vi "MListbox Clear All Rows.vi"(8 "error in (no error)":errorcluster, 11 "Multicolumn ListBox in":refnum<class "Multicolumn ListBox.lvclass">) -> (0 "error out":errorcluster, 3 "Multicolumn ListBox out":refnum<class "Multicolumn ListBox.lvclass">)   [LabVIEW 2012, in "Multicolumn ListBox.lvclass"]
uses:
  Multicolumn ListBox.lvclass
  <vilib>/Utility/miscctls.llb/LVRowAndColumnUnsignedTypeDef.ctl
  <vilib>/Utility/miscctls.llb/LVRowAndColumnTypeDef.ctl
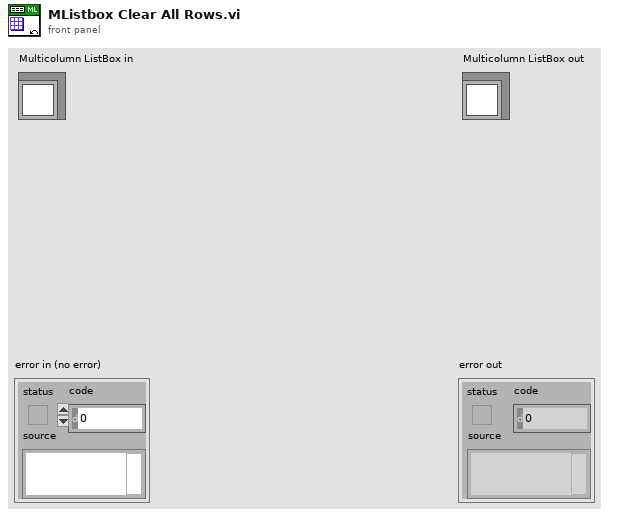
[diagram p1: front panel]
types:
  T1 = typedef "LVRowAndColumnTypeDef.ctl" = cluster{"Row":i32, "Column":i32}
  T2 = typedef "LVRowAndColumnUnsignedTypeDef.ctl" = cluster{"Row":u32, "Column":u32}
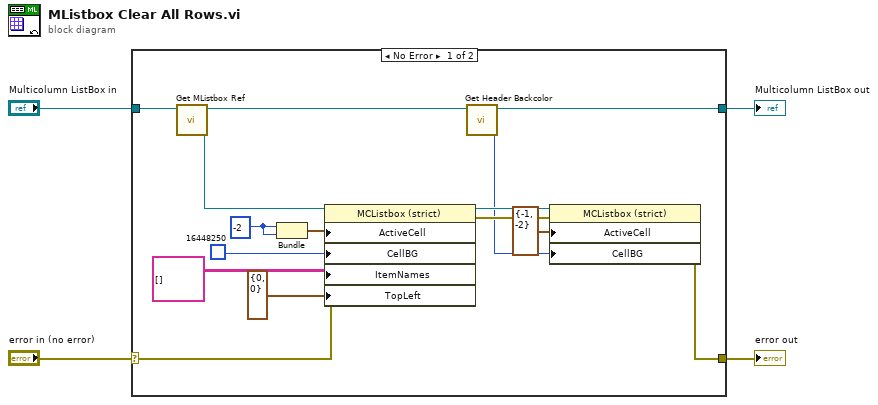
[diagram p0: block diagram]
diagram:
  n1 = case shown="No Error" "error in (no error)" {
    selector: "error in (no error)" -> [w12 w21]
    tunnel: [w7 w21] -> w3
    tunnel: [w17 w20] -> w1
    tunnel: "Multicolumn ListBox in" -> [w19 w20]
    frame No Error {
      w16 = -2
      n2 = call "Get MListbox Ref.vi"("Multicolumn ListBox in"=w19) -> ("MListbox Ref"=w13:refnum<vi>, "Multicolumn ListBox out"=w18:refnum<class "Multicolumn ListBox.lvclass">)  [unwired: 8 in, 1 out]
      n3 = Bundle(w16, w16) -> (w15:cluster{i32, i32})  [unwired: 1 in]
      n4 = property class="MCListbox (strict)"(reference=w13, error in=w12, "ActiveCell"=w15, "CellBG"=u32 16448250, "ItemNames"=string[][] [] ("Item Names"), "TopLeft"=T2 {"Row"=0, "Column"=0} ("Top Left Visible Cell")) -> (reference out=w9:refnum<vi>, error out=w8:errorcluster)
      n5 = call "Get Header Backcolor.vi"("Multicolumn ListBox in"=w18) -> ("Header Backcolor"=w6:u32, "Multicolumn ListBox out"=w17:refnum<class "Multicolumn ListBox.lvclass">)  [unwired: 8 in, 1 out]
      n6 = property class="MCListbox (strict)"(reference=w9, error in=w8, "ActiveCell"=T1 {"Row"=-1, "Column"=-2} ("Active Cell:Active Cell"), "CellBG"=w6) -> (error out=w7:errorcluster)  [unwired: 1 out]
    }
    frame Error {
    }
  }
  "error out" <- w3
  "Multicolumn ListBox out" <- w1
